vi "Read_Exposures.vi"(6 "ref in":i32, 7 "sequencer":T1(array[cluster]), 8 "error in":errorcluster) -> (0 "ref out":i32, 1 "ROI":T2, 2 "loaded images":u16[][][](array[numeric]), 4 "computations":T3(array[cluster]), 5 "error out":errorcluster)   [LabVIEW 2010]
uses:
  <userlib>/bias/subvis/ROI_rect.ctl
  <vilib>/addons/h5labview2/attrib/H5Aread.llb/H5Aread.xnode
  <vilib>/addons/h5labview2/base/hid_t.ctl
  <vilib>/addons/h5labview2/dataset/H5Dread.llb/H5Dread.xnode
  <vilib>/addons/h5labview2/base/lib_path.vi
  <vilib>/addons/h5labview2/base/H5Equery.vi
  <vilib>/addons/h5labview2/group/H5G.lvlib
  <vilib>/addons/h5labview2/type/H5T.lvlib
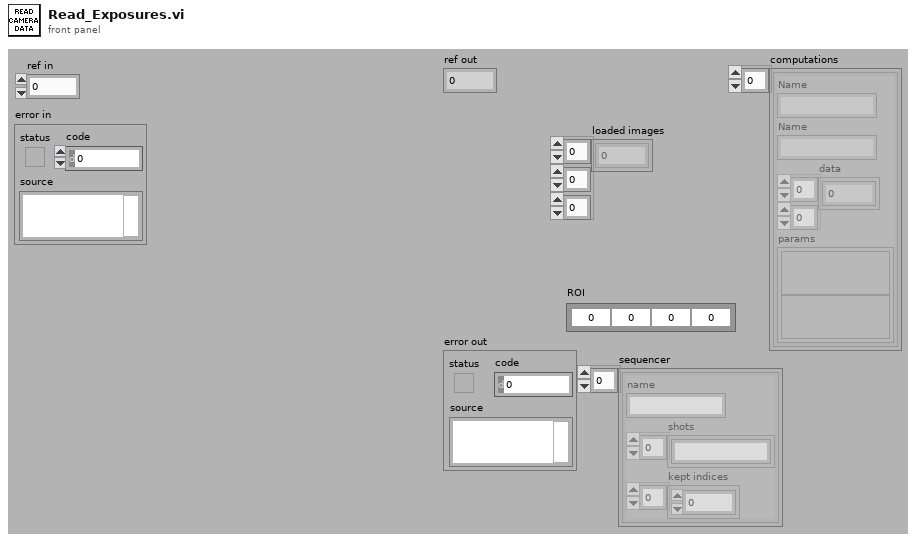
[diagram p1: front panel]
types:
  T1 = cluster{"name":string, "shots":string[], "kept indices":i32[]}[]
  T2 = typedef "ROI_rect.ctl" = cluster{"left":i32, "top":i32, "right":i32, "bottom":i32}
  T3 = cluster{"Name":string, "Name":string, "data":sgl[][], "params":variant[]}[]
  T4 = typedef "hid_t.ctl" = i32
  T5 = cluster{"name":string, "shots":string[], "kept indices":i32[]}
  T6 = typedef "h5o_type.ctl" = enum8{"Group", "Dataset", "Named type"}
  T7 = typedef "hclass_t.ctl" = enum16{"H5T_INTEGER", "H5T_FLOAT", "H5T_TIME", "H5T_STRING", "H5T_BITFIELD", "H5T_OPAQUE", "H5T_COMPOUND", "H5T_REFERENCE", "H5T_ENUM", "H5T_VLEN", "H5T_ARRAY"}
  T8 = cluster{"name":string, "name":string, "data":sgl[][], variant[]}
  T9 = cluster{"name":string, "name":string, "data":sgl[][], "params":variant[]}[]
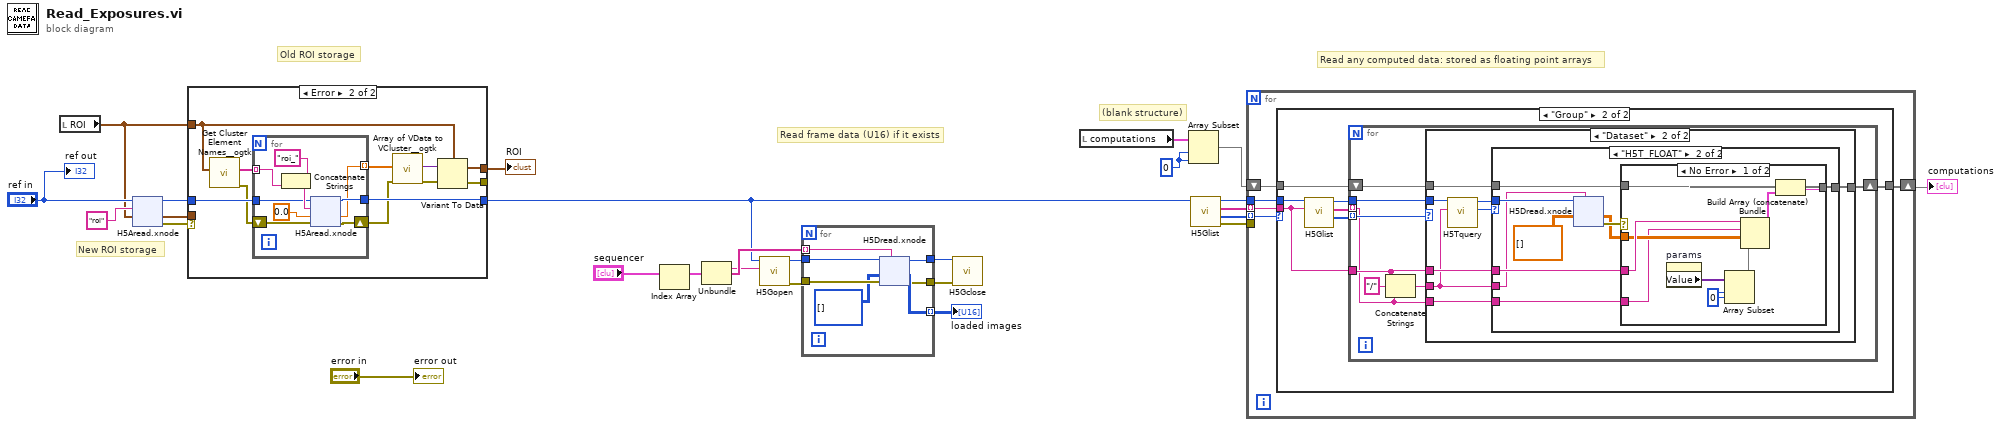
[diagram p0: block diagram]
diagram:
  w23 = 0 ("length")
  # "(blank structure)"
  # "Old ROI storage"
  # "New ROI storage"
  # "Read any computed data: stored as floating point arrays"
  # "Read frame data (U16) if it exists"
  n1 = local read "ROI"() -> (w13:T2)
  n2 = xnode "H5Aread.xnode"("default"=w13, "attrib name"="roi" ("prefix"), "ref in"="ref in") -> ("error out"=w11:errorcluster, "data"=w10:T2, "ref out"=w12:T4)  [unwired: 3 in, 1 out]
  n3 = case shown="Error" w11 {
    tunnel: w13 -> [_ w34]
    tunnel: w12 -> [w27 w37]
    tunnel: [w26 w29] -> w21
    tunnel: [w27 w36] -> w3
    tunnel: [_ w28] -> _
    tunnel: w10 -> [w26 _]
    frame No Error {
    }
    frame Error {
      n4 = call <userlib>:"Get Cluster Element Names__ogtk.vi"("Cluster"=w34) -> ("error out"=w35:errorcluster, "Element Names"=w38:string[])  [unwired: 9 in]
      n5 = for {
        tunnel: w38 -> [w46] mode=indexing
        tunnel: w37 -> [w44]
        tunnel: [w41] -> w36
        shift-right: [w42] -> w32
        shift-left: w35 -> [w43]
        tunnel: [w39] -> w33 mode=indexing
        n6 = Concatenate Strings("roi_" ("prefix"), w46) -> (w45:string)
        n7 = xnode "H5Aread.xnode"("error in (no error)"=w43, "default"=0.0, "attrib name"=w45, "ref in"=w44) -> ("error out"=w42:errorcluster, "data"=w39:dbl, "ref out"=w41:T4)  [unwired: 2 in, 1 out]
      }
      n8 = call <userlib>:"Array of VData to VCluster__ogtk.vi"("error in (no error)"=w32, "Array"=w33) -> ("error out"=w31:errorcluster, "VCluster"=w30:variant)  [unwired: 8 in]
      n9 = Variant To Data(error in=w31, Variant=w30, type=w34) -> (error out=w28:errorcluster, data=w29:T2)
    }
  }
  "ROI" <- w21
  n10 = Index Array(array="sequencer") -> (element=w17:T5)  [unwired: 1 in]
  n11 = Unbundle(w17) -> ("name"=w9:string, "shots"=w18:string[])  [unwired: 1 out]
  n12 = call <vilib>:"H5Gopen.vi"("name"=w9, "ref in"=w3) -> ("error out"=w7:errorcluster, "group out"=w8:T4)  [unwired: 8 in]
  n13 = for {
    tunnel: w8 -> [w69]
    tunnel: w18 -> [w67] mode=indexing
    tunnel: w7 -> [w68]
    tunnel: [w65] -> w6
    tunnel: [w66] -> w16 mode=indexing
    tunnel: [w63] -> w5
    n14 = xnode "H5Dread.xnode"("dataset name (this)"=w67, "error in (no error)"=w68, "default"=u16[][] [], "ref in"=w69) -> ("error out"=w65:errorcluster, "data"=w66:u16[][], "ref out"=w63:T4)  [unwired: 2 in, 1 out]
  }
  "loaded images" <- w16
  n15 = call <vilib>:"H5Gclose.vi"("error in (no error)"=w6, "group in"=w5) -> ()  [unwired: 9 in, 1 out]
  n16 = local read "computations"() -> (w24:T3)
  n17 = Array Subset(array=w24, index=w23, length=w23) -> (w22:T3)
  n18 = call <vilib>:"H5Glist.vi"("ref in"=w3) -> ("error out"=w4:errorcluster, "types"=w1:T6[], "names"=w2:string[])  [unwired: 7 in, 1 out]
  n19 = for {
    shift-right: [w88] -> w25
    shift-left: w22 -> [w89]
    tunnel: w3 -> [w86]
    tunnel: w2 -> [w85] mode=indexing
    tunnel: w1 -> [w87] mode=indexing
    tunnel: w4 -> [_]
    n20 = case shown="\"Group\"" w87 {
      tunnel: w89 -> [w90 w97]
      tunnel: [w90 w96] -> w88
      tunnel: w86 -> [_ w95]
      tunnel: w85 -> [_ w91]
      frame Default {
      }
      frame "Group" {
        n21 = call <vilib>:"H5Glist.vi"("group (.)"=w91, "ref in"=w95) -> ("types"=w92:T6[], "names"=w93:string[], "ref out"=w94:T4)  [unwired: 6 in, 1 out]
        n22 = for {
          shift-right: [w104] -> w96
          shift-left: w97 -> [w105]
          tunnel: w94 -> [w98]
          tunnel: w93 -> [w100] mode=indexing
          tunnel: w92 -> [w103] mode=indexing
          tunnel: w91 -> [w101]
          n23 = Concatenate Strings(w101, "/" ("string"), w100) -> (w99:string)
          n24 = case shown="\"Dataset\"" w103 {
            tunnel: w105 -> [w106 w114]
            tunnel: [w106 w113] -> w104
            tunnel: w101 -> [_ w112]
            tunnel: w100 -> [_ w111]
            tunnel: w99 -> [_ w108]
            tunnel: w98 -> [_ w110]
            frame Default {
            }
            frame "Dataset" {
              n25 = call <vilib>:"H5Tquery.vi"("obj name"=w108, "ref in"=w110) -> ("class"=w107:T7, "ref out"=w109:T4)  [unwired: 4 in, 4 out]
              n26 = case shown="\"H5T_FLOAT\"" w107 {
                tunnel: w114 -> [w115 w124]
                tunnel: [w115 w123] -> w113
                tunnel: w112 -> [_ w122]
                tunnel: w109 -> [_ w120]
                tunnel: w111 -> [_ w121]
                tunnel: w108 -> [_ w118]
                frame Default {
                }
                frame "H5T_FLOAT" {
                  n27 = xnode "H5Dread.xnode"("dataset name (this)"=w118, "default"=sgl[][] [], "ref in"=w120) -> ("error out"=w119:errorcluster, "data"=w117:sgl[][])  [unwired: 3 in, 2 out]
                  n28 = case shown="No Error" w119 {
                    tunnel: w124 -> [w148 w149]
                    tunnel: [w147 w149] -> w123
                    tunnel: w117 -> [w142 _]
                    tunnel: w122 -> [w143 _]
                    tunnel: w121 -> [w141 _]
                    frame No Error {
                      w144 = 0 ("length")
                      n29 = property on="params" class="Arr (strict)"() -> ("Value"=w146:variant[])  [unwired: 2 in, 2 out]
                      n30 = Array Subset(array=w146, index=w144, length=w144) -> (w145:variant[])
                      n31 = Bundle("name"=w143, "name"=w141, "data"=w142, w145) -> (w140:T8)  [unwired: 1 in]
                      n32 = Build Array (concatenate)(w148, w140) -> (w147:T9)
                    }
                    frame Error {
                    }
                  }
                }
              }
            }
          }
        }
      }
    }
  }
  "computations" <- w25
  "error out" <- "error in"
  "ref out" <- "ref in"
